vi "Neo-T.vi"(2 "Where? Forebrain":cluster{"T":dbl, "X":dbl, "Y":dbl}, 5 "What?Forebrain":cluster{"T":dbl, "Range":dbl, "Bearing":dbl}[](array[cluster])) -> (1 "Act Forebrain":cluster{"Motor1":i16, "Motor 2":i16})   [LabVIEW 2010]
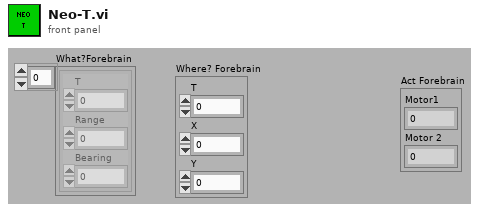
[diagram p1: front panel]
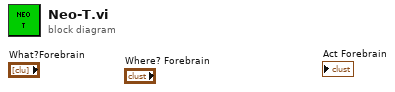
[diagram p0: block diagram]
diagram:
